vi "DSF.Engine.Transceiver.Tx.vi"(8 "error in (no error)":errorcluster, 10 "Transfer Group in":refnum<class "DSF.Engine.Transfer Group.lvclass">, 11 "Transceiver in":refnum<class "DSF.Transceiver.UDP.lvclass">) -> (0 "error out":errorcluster, 2 "Transfer Group out":refnum<class "DSF.Engine.Transfer Group.lvclass">, 3 "Transceiver out":refnum<class "DSF.Transceiver.UDP.lvclass">)   [LabVIEW 2017, in "DSF.Transceiver.UDP.lvlib" / "DSF.Transceiver.UDP.lvclass"]
uses:
  DSF.Transceiver.UDP.lvclass
  Built/Windows/Engine/DSF.Engine.lvlibp/Engine/Classes/Transfer/DSF.Engine.Transfer Group.lvclass
  DSF.Transceiver.UDP.lvclass/DSF.Transceiver.UDP.ctl
  Built/Windows/Engine/DSF.Engine.lvlibp/Engine/Classes/Buffer/DSF.Engine.Memory.Buffer.Read.1D.U8.vi
  Built/Windows/Engine/DSF.Engine.lvlibp/Engine/Classes/Transfer/DSF.Engine.Transfer.lvclass
  Built/Windows/Engine/DSF.Engine.lvlibp/Engine/Classes/Buffer/DSF.Engine.Memory.Buffer.lvclass
  Built/Windows/Dependencies/Memory Manager.lvlibp/1abvi3w/vi.lib/National Instruments/Memory Manager/Classes/Pointer/Memory.Pointer.lvclass
  C:/Git/DSF/dsf core/Built/Windows/Dependencies/Memory Manager.lvlibp/1abvi3w/vi.lib/National Instruments/Memory Manager/Classes/Pointer/Memory.Pointer.lvclass
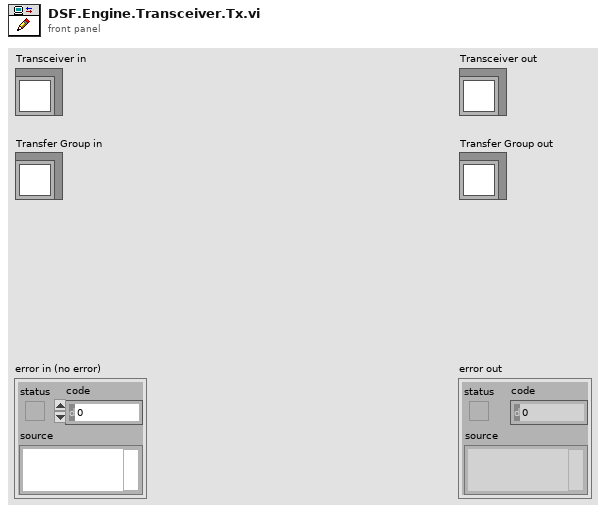
[diagram p1: front panel]
types:
  T1 = typedef "DSF.Transceiver.UDP.lvlib/DSF.Transceiver.UDP.lvclass/DSF.Transceiver.UDP.Tx Parameters.ctl" = cluster{"connection ID":refnum<k16>, "address":u32, "port or service name":u16}
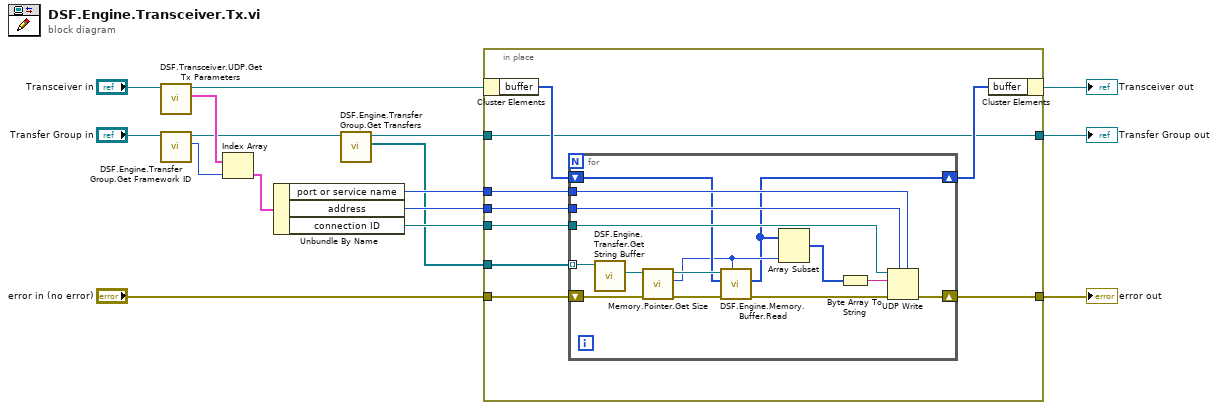
[diagram p0: block diagram]
diagram:
  n1 = call "DSF.Transceiver.UDP.Get Tx Parameters.vi"("DSF.Transceiver.UDP in"="Transceiver in") -> ("Tx parameters"=w16:T1[], "DSF.Transceiver.UDP out"=w4:refnum<class "DSF.Transceiver.UDP.lvclass">)  [unwired: 9 in]
  n2 = call "DSF.Engine.Transfer Group.Get Framework ID.vi"("Transfer Group in"="Transfer Group in") -> ("framework id"=w15:i32, "Transfer Group out"=w12:refnum<class "DSF.Engine.Transfer Group.lvclass">)  [unwired: 9 in]
  n3 = Index Array(array=w16, index=w15) -> (element=w14:T1)
  n4 = Unbundle By Name(w14) -> ("port or service name"=w10:u16, "address"=w11:u32, "connection ID"=w13:refnum<k16>)
  n5 = call "DSF.Engine.Transfer Group.Get Transfers.vi"("Transfer Group in"=w12) -> ("Transfers"=w9:refnum<class "DSF.Engine.Transfer.lvclass">[], "Transfer Group out"=w2:refnum<class "DSF.Engine.Transfer Group.lvclass">)  [unwired: 9 in]
  n6 = in-place {
    in-place-border: w13 -> [w25]
    in-place-border: w11 -> [w24]
    in-place-border: w10 -> [w23]
    in-place-border: w9 -> [w22]
    in-place-border: "error in (no error)" -> [w21]
    in-place-border: [w20] -> w5
    in-place-border: w2 -> [w17]
    in-place-border: [w17] -> w1
    n7 = in-place-cluster #1(w4) -> ("buffer"=w19:u8[])
    n8 = for {
      tunnel: w25 -> [w38]
      shift-right: [w39] -> w20
      shift-left: w21 -> [w36]
      tunnel: w22 -> [w37] mode=indexing
      tunnel: w24 -> [w31]
      tunnel: w23 -> [w30]
      shift-right: [w27] -> w18
      shift-left: w19 -> [w29]
      n9 = call "DSF.Engine.Transfer.Get String Buffer.vi"("Transfer in"=w37) -> ("Buffer"=w34:refnum<class "DSF.Engine.Memory.Buffer.lvclass">)  [unwired: 9 in, 1 out]
      n10 = call "Memory.Pointer.Get Size.vi"("Pointer in"=w34) -> ("size"=w28:u64, "Pointer out"=w33:refnum<class "DSF.Engine.Memory.Buffer.lvclass">)  [unwired: 9 in]
      n11 = call-poly "DSF.Engine.Memory.Buffer.Read.vi"("count"=w28, "error in (no error)"=w36, "buffer in"=w29, "Buffer in"=w33) -> ("error out"=w35:errorcluster, "buffer out"=w27:u8[])  [unwired: 4 in, 2 out]
      n12 = Array Subset(array=w27, length=w28) -> (w26:u8[])  [unwired: 1 in]
      n13 = Byte Array To String(unsigned byte array=w26) -> (string=w32:string)
      n14 = UDP Write(address=w31, port or service name=w30, connection ID=w38, data in=w32, 8:w35) -> (error out=w39:errorcluster)  [unwired: 1 in, 1 out]
    }
    n15 = in-place-cluster #1("buffer"=w18) -> (→"Transceiver out":refnum<class "DSF.Transceiver.UDP.lvclass">)
  }
  "error out" <- w5
  "Transfer Group out" <- w1
